vi "Initialize.vi"(0 "Noise in":refnum<class "Noise.lvclass">, 1 "Filter in":refnum<class "Filter.lvclass">, 5 "Level in":refnum<class "Level.lvclass">, 7 "Fs (Hz)":dbl, 9 "Npts":i32, 11 "error in (no error)":errorcluster, 13 "Channel Name":string) -> (3 "Filter out":refnum<class "Filter.lvclass">, 4 "Noise out":refnum<class "Noise.lvclass">, 6 "Level out":refnum<class "Level.lvclass">, 15 "error out":errorcluster)   [LabVIEW 2020, in "Noise.lvclass"]
uses:
  Noise.lvclass
  Level/Level.lvclass
  Filter/Filter.lvclass
  Noise.lvclass/Noise.ctl
  Filter/Filter.lvclass/Filter.ctl
  Filter/Read Type.vi
  Filter/Read Class.vi
  <vilib>/Analysis/NI_AALBase.lvlib
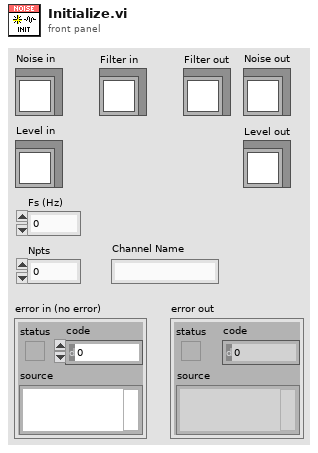
[diagram p1: front panel]
types:
  T1 = enum16{"Clear", "Set data", "Reset index", "Get data"}
  T2 = typedef "Filter.lvclass/Shape.ctl" = enum16{"OFF", "Lowpass", "Highpass", "Bandpass", "Bandstop"}
  T3 = typedef "Filter.lvclass/Class.ctl" = enum16{"Elliptic", "Butterworth", "Brickwall"}
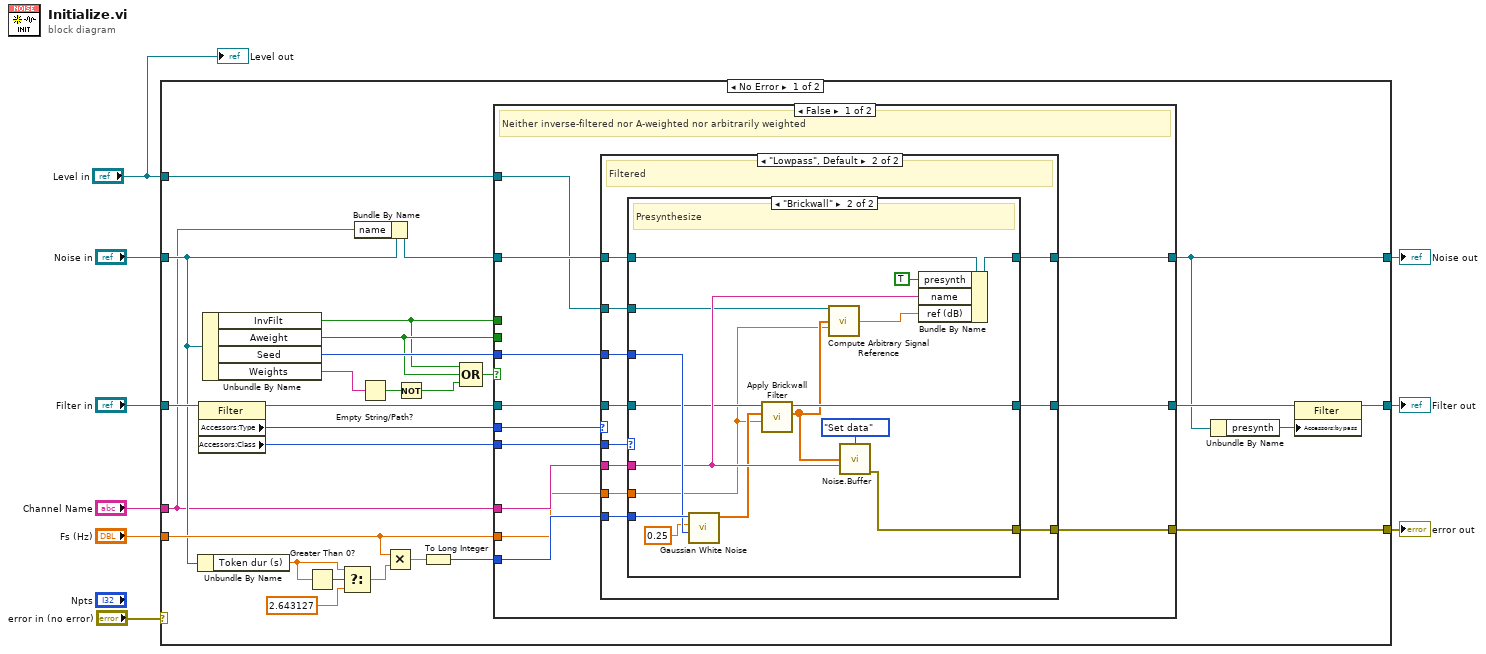
[diagram p0: block diagram]
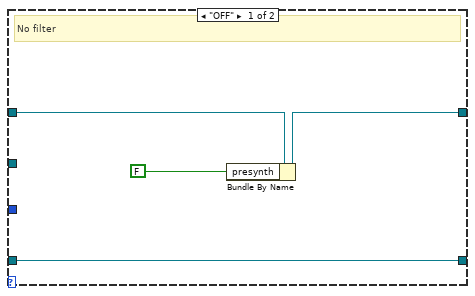
[diagram p2: hidden frame]
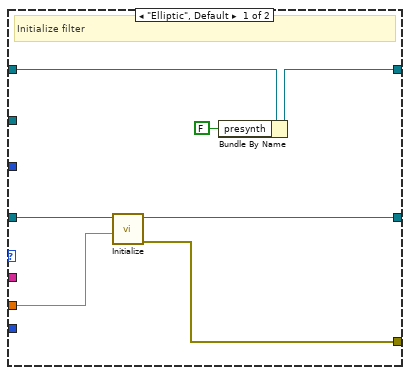
[diagram p3: hidden frame]
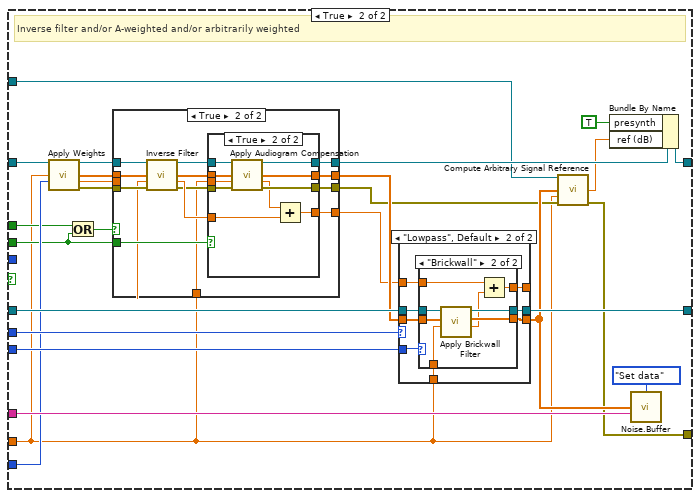
[diagram p4: hidden frame]
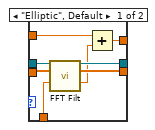
[diagram p8: hidden frame]
diagram:
  n1 = case shown="No Error" "error in (no error)" {
    selector: "error in (no error)" -> [_ w173]
    tunnel: "Noise in" -> [w27 w172]
    tunnel: [w36 w173] -> w8
    tunnel: [w11 w172] -> w7
    tunnel: "Filter in" -> [w35 w171]
    tunnel: [w13 w171] -> w5
    tunnel: "Fs (Hz)" -> [w28 _]
    tunnel: "Channel Name" -> [w21 _]
    tunnel: "Level in" -> [w14 _]
    frame No Error {
      n2 = Unbundle By Name(w27) -> ("Token dur (s)"=w25:dbl)
      n3 = property class="Filter"(reference=w35) -> (reference out=w33:refnum<class "Filter.lvclass">, "Accessors:Type"=w34:T2, "Accessors:Class"=w32:T3)  [unwired: 1 in, 1 out]
      n4 = Unbundle By Name(w27) -> ("InvFilt"=w17:bool, "Aweight"=w18:bool, "Seed"=w29:i32, "Weights"=w15:string)
      n5 = Greater Than 0?(x=w25) -> (x > 0?=w26:bool)
      n6 = Select(t=w25, s=w26, f=2.643127) -> (s? t:f=w23:dbl)
      n7 = Bundle By Name(cluster=w27, "name"=w21) -> (w22:refnum<class "Noise.lvclass">)
      n8 = Empty String/Path?(string/path=w15) -> (empty?=w20:bool)
      n9 = Multiply(x=w28, y=w23) -> (x*y=w31:dbl)
      n10 = Not(x=w20) -> (.not. x?=w16:bool)
      n11 = To Long Integer(number=w31) -> (32bit integer=w30:i32)
      n12 = Compound Arithmetic op=OR(w17, w18, w16) -> (w19:bool)
      n13 = case shown="False" w19 {
        tunnel: [w42 w89] -> w36
        tunnel: w22 -> [w46 w101]
        tunnel: [w47 w112] -> w11
        tunnel: w34 -> [w48 w108]
        tunnel: [w45 w105] -> w12
        tunnel: w33 -> [w44 w106]
        tunnel: w32 -> [w43 w107]
        tunnel: w30 -> [w41 w98]
        tunnel: w29 -> [w40 _]
        tunnel: w21 -> [w39 w109]
        tunnel: w28 -> [w38 w87]
        tunnel: w18 -> [_ w96]
        tunnel: w17 -> [_ w97]
        tunnel: w14 -> [w37 w91]
        frame False {
          # "Neither inverse-filtered nor A-weighted nor arbitrarily weighted"
          n14 = case shown="\"Lowpass\", Default" w48 {
            tunnel: [w50 w62] -> w47
            tunnel: w46 -> [w52 w61]
            tunnel: [w51 w60] -> w45
            tunnel: w44 -> [w51 w59]
            tunnel: w43 -> [_ w63]
            tunnel: [_ w58] -> w42
            tunnel: w41 -> [_ w57]
            tunnel: w40 -> [_ w56]
            tunnel: w39 -> [_ w55]
            tunnel: w38 -> [_ w54]
            tunnel: w37 -> [_ w53]
            frame "OFF" {
              # "No filter"
              n15 = Bundle By Name(cluster=w52, "presynth"=FALSE) -> (w50:refnum<class "Noise.lvclass">)
            }
            frame "Lowpass", Default {
              # "Filtered"
              n16 = case shown="\"Brickwall\"" w63 {
                tunnel: [w69 w85] -> w62
                tunnel: w61 -> [w70 w86]
                tunnel: [w66 w76] -> w60
                tunnel: w59 -> [w67 w77]
                tunnel: [w65 w78] -> w58
                tunnel: w57 -> [_ w83]
                tunnel: w56 -> [_ w82]
                tunnel: w55 -> [_ w79]
                tunnel: w54 -> [w64 w71]
                tunnel: w53 -> [_ w72]
                frame "Elliptic", Default {
                  # "Initialize filter"
                  n17 = call "Initialize.vi"("Fs (Hz)"=w64, "Filter in"=w67) -> ("error out"=w65:errorcluster, "Filter out"=w66:refnum<class "Filter.lvclass">)  [unwired: 8 in]
                  n18 = Bundle By Name(cluster=w70, "presynth"=FALSE) -> (w69:refnum<class "Noise.lvclass">)
                }
                frame "Brickwall" {
                  # "Presynthesize"
                  n19 = call <vilib>:"Gaussian White Noise.vi"("seed"=w82, "standard deviation"=0.25, "samples"=w83) -> ("Gaussian noise pattern"=w75:dbl[])  [unwired: 7 in, 1 out]
                  n20 = call "Apply Brickwall Filter.vi"("Fs (Hz)"=w71, "Signal In"=w75, "Filter in"=w77) -> ("Signal Out"=w74:dbl[], "Filter out"=w76:refnum<class "Filter.lvclass">)  [unwired: 5 in, 2 out]
                  n21 = call "Compute Arbitrary Signal Reference.vi"("Level in"=w72, "signal"=w74, "Fs"=w71) -> ("ref"=w73:dbl)  [unwired: 10 in, 2 out]
                  n22 = call "Noise.Buffer.vi"("Action"=T1."Set data", "Data In"=w74, "Name"=w79) -> ("error out"=w78:errorcluster)  [unwired: 11 in, 1 out]
                  n23 = Bundle By Name(cluster=w86, "presynth"=TRUE, "name"=w79, "ref (dB)"=w73) -> (w85:refnum<class "Noise.lvclass">)
                }
              }
            }
          }
        }
        frame True {
          # "Inverse filter and/or A-weighted and/or arbitrarily weighted"
          n24 = call "Apply Weights.vi"("Noise in"=w101, "Fs (Hz)"=w87, "Npts"=w98) -> ("Noise out"=w100:refnum<class "Noise.lvclass">, "noise"=w95:dbl[], "reference"=w93:dbl, "error out"=w99:errorcluster)  [unwired: 9 in]
          n25 = Or(x=w97, y=w96) -> (x .or. y?=w94:bool)
          n26 = case shown="True" w94 {
            tunnel: [w116 w129] -> w104
            tunnel: [w115 w127] -> w103
            tunnel: [w113 w123] -> w102
            tunnel: [w114 w122] -> w90
            tunnel: w100 -> [w116 w121]
            tunnel: w99 -> [w114 w120]
            tunnel: w96 -> [_ w119]
            tunnel: w95 -> [w115 w118]
            tunnel: w87 -> [_ w117]
            tunnel: w93 -> [w113 _]
            frame False {
            }
            frame True {
              n27 = call "Inverse Filter.vi"("Noise in"=w121, "noise in"=w118, "Fs (Hz)"=w117, "error in (no error)"=w120) -> ("Noise out"=w128:refnum<class "Noise.lvclass">, "noise out"=w126:dbl[], "reference"=w125:dbl, "error out"=w124:errorcluster)  [unwired: 8 in]
              n28 = case shown="True" w119 {
                tunnel: [w133 w142] -> w129
                tunnel: w128 -> [w133 w143]
                tunnel: [w132 w141] -> w127
                tunnel: w126 -> [w132 w140]
                tunnel: w125 -> [w130 w136]
                tunnel: w124 -> [w131 w139]
                tunnel: [w131 w138] -> w122
                tunnel: [w130 w134] -> w123
                tunnel: w117 -> [_ w137]
                frame False {
                }
                frame True {
                  n29 = call "Apply Audiogram Compensation.vi"("Noise in"=w143, "Noise (flattened!)"=w140, "Fs (Hz)"=w137, "error in (no error)"=w139) -> ("Noise out"=w142:refnum<class "Noise.lvclass">, "Compensated"=w141:dbl[], "Gain"=w135:dbl, "error out"=w138:errorcluster)  [unwired: 8 in]
                  n30 = Add(x=w135, y=w136) -> (x+y=w134:dbl)
                }
              }
            }
          }
          n31 = case shown="\"Lowpass\", Default" w108 {
            tunnel: w103 -> [w145 w151]
            tunnel: w102 -> [w144 w148]
            tunnel: w107 -> [_ w154]
            tunnel: w106 -> [w146 w153]
            tunnel: [w146 w152] -> w105
            tunnel: w87 -> [_ w150]
            tunnel: [w145 w149] -> w92
            tunnel: [w144 w147] -> _
            frame "OFF" {
            }
            frame "Lowpass", Default {
              n32 = case shown="\"Brickwall\"" w154 {
                tunnel: w153 -> [w162 w170]
                tunnel: [w160 w169] -> w152
                tunnel: w151 -> [w161 w168]
                tunnel: w150 -> [w158 w167]
                tunnel: [w159 w166] -> w149
                tunnel: w148 -> [w157 w165]
                tunnel: [w156 w163] -> w147
                frame "Elliptic", Default {
                  n33 = call "FFT Filt.vi"("Filter in"=w162, "Y"=w161, "Fs (Hz)"=w158) -> ("Filter out"=w160:refnum<class "Filter.lvclass">, "Yfilt"=w159:dbl[], "Gain"=w155:dbl)  [unwired: 9 in, 1 out]
                  n34 = Add(x=w157, y=w155) -> (x+y=w156:dbl)
                }
                frame "Brickwall" {
                  n35 = call "Apply Brickwall Filter.vi"("Fs (Hz)"=w167, "Signal In"=w168, "Filter in"=w170) -> ("Gain (dB)"=w164:dbl, "Signal Out"=w166:dbl[], "Filter out"=w169:refnum<class "Filter.lvclass">)  [unwired: 5 in, 1 out]
                  n36 = Add(x=w165, y=w164) -> (x+y=w163:dbl)
                }
              }
            }
          }
          n37 = call "Compute Arbitrary Signal Reference.vi"("Level in"=w91, "signal"=w92, "Fs"=w87, "error in (no error)"=w90) -> ("ref"=w88:dbl, "error out"=w89:errorcluster)  [unwired: 9 in, 1 out]
          n38 = Bundle By Name(cluster=w104, "presynth"=TRUE, "ref (dB)"=w88) -> (w112:refnum<class "Noise.lvclass">)
          n39 = call "Noise.Buffer.vi"("Action"=T1."Set data", "Data In"=w92, "Name"=w109) -> ()  [unwired: 11 in, 2 out]
        }
      }
      n40 = Unbundle By Name(w11) -> ("presynth"=w10:bool)
      n41 = property class="Filter"(reference=w12, "Accessors:bypass"=w10) -> (reference out=w13:refnum<class "Filter.lvclass">)  [unwired: 1 in, 1 out]
    }
    frame Error {
    }
  }
  "error out" <- w8
  "Noise out" <- w7
  "Filter out" <- w5
  "Level out" <- "Level in"
